vi "GetTimeInSeconds.vi"(11 "Timestamp":timestamp) -> (3 "Numeric":dbl)   [LabVIEW 2017]
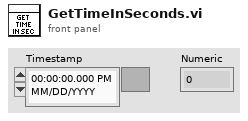
[diagram p1: front panel]
types:
  T1 = typedef "LVDateTimeRec.ctl" = cluster{"fractional second":dbl, "second":i32, "minute":i32, "hour":i32, "day of month":i32, "month":i32, "year":i32, "day of week":i32, "day of year":i32, "DST":i32}
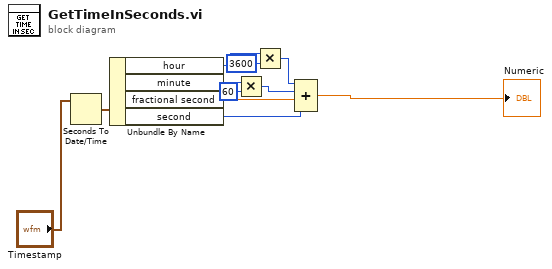
[diagram p0: block diagram]
diagram:
  n1 = Seconds To Date/Time(time stamp (now)="Timestamp") -> (date time rec=w1:T1)  [unwired: 1 in]
  n2 = Unbundle By Name(w1) -> ("hour"=w8:i32, "minute"=w4:i32, "fractional second"=w2:dbl, "second"=w3:i32)
  n3 = Multiply(x=w4, y=60) -> (x*y=w6:i32)
  n4 = Multiply(x=w8, y=3600) -> (x*y=w9:i32)
  n5 = Compound Arithmetic op=ADD(w9, w6, w2, w3) -> (→"Numeric":dbl)
